vi "Продукты 2022.vi"() -> ()   [LabVIEW 2020]
uses:
  Control 2.ctl
panel:
  out "Array":T1[](array[typedef]) {"T" scale=-20.0..40.0; "Time Stamp" format="%<%2d/%2m/%4Y>T"}
  in  "Купить":bool
  in  "Покупаемый продукт":T1 {"T" scale=-20.0..40.0; "Time Stamp" format="%<%2d/%2m/%4Y>T"}
  in  "stop":bool
  out "String":string
  in  "Добавить":bool
  in  "Добавляемый продукт":T1 {"T" scale=-20.0..40.0; "Time Stamp" format="%<%2d/%2m/%4Y>T"}
  # "Прибыль магазина"
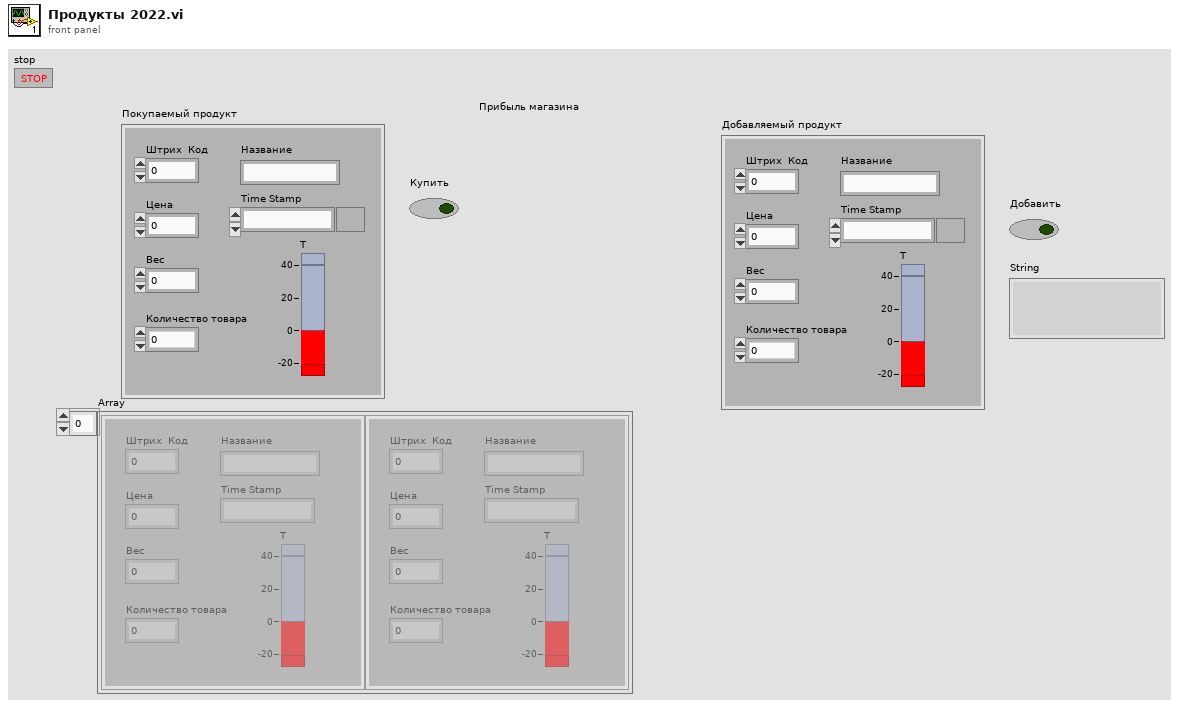
[diagram p1: front panel]
types:
  T1 = typedef "Control 2.ctl" = cluster{"Штрих  Код":dbl, "Цена":dbl, "Название":string, "Time Stamp":timestamp, "Вес":dbl, "T":dbl, "Количество товара":dbl}
  T2 = cluster{"Штрих  Код":dbl, "Цена":dbl, "Название":string, "Time Stamp":timestamp, "Вес":dbl, "T":dbl, "T 2":dbl}[]
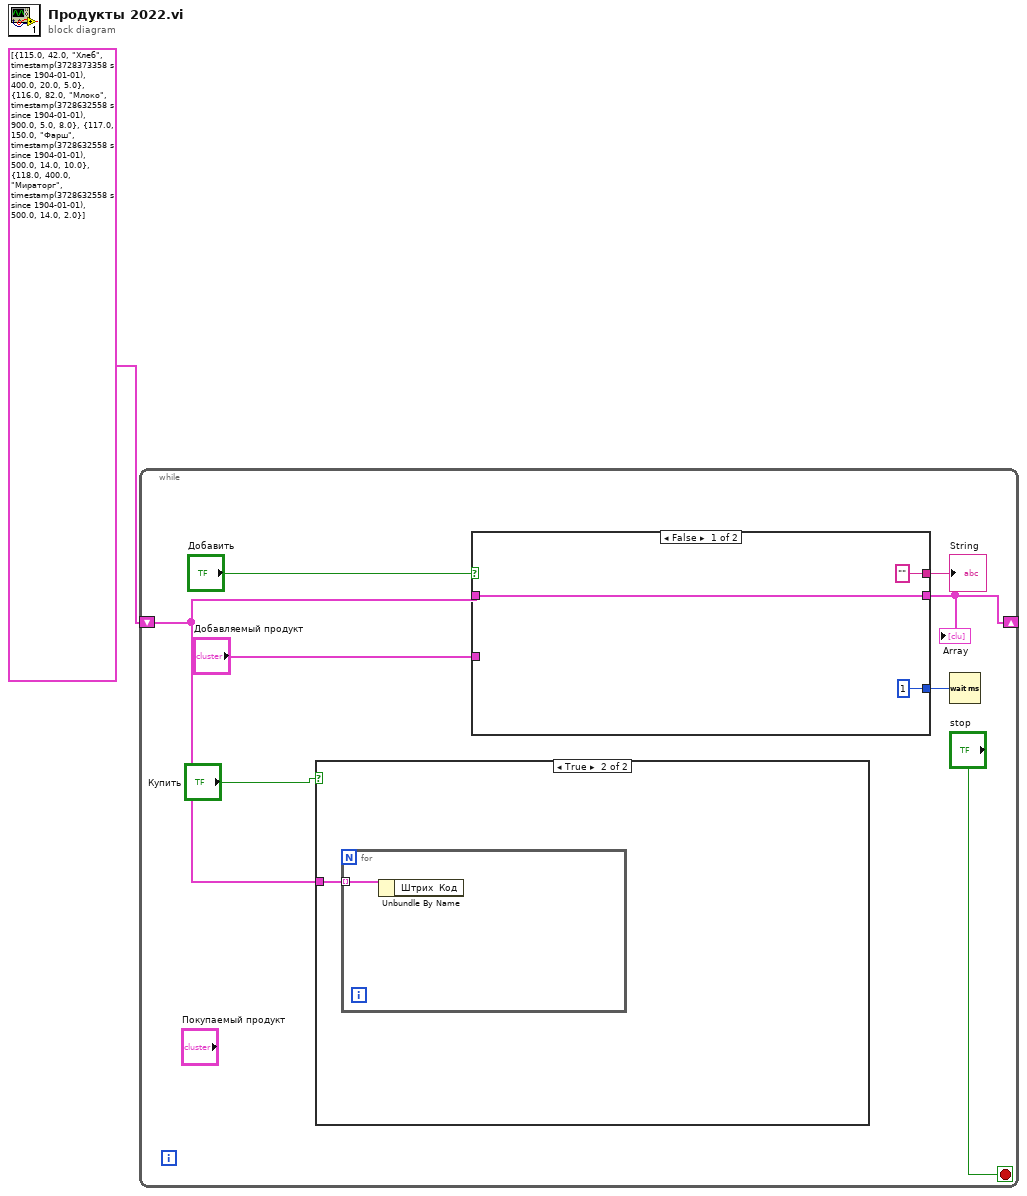
[diagram p0: block diagram]
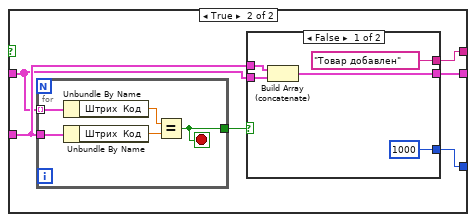
[diagram p3: hidden frame]
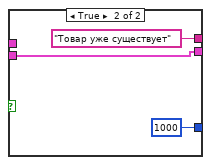
[diagram p4: hidden frame]
diagram:
  n1 = while {
    shift-right: [w2] -> _
    shift-left: T2 [{"Штрих  Код"=115.0, "Цена"=42.0, "Название"="Хлеб", "Time Stamp"=timestamp(3728373358.5762897 s since 1904-01-01), "Вес"=400.0, "T"=20.0, "T 2"=5.0}, {"Штрих  Код"=116.0, "Цена"=82.0, "Название"="Млоко", "Time Stamp"=timestamp(3728632558.5762897 s since 1904-01-01), "Вес"=900.0, "T"=5.0, "T 2"=8.0}, {"Штрих  Код"=117.0, "Цена"=150.0, "Название"="Фарш", "Time Stamp"=timestamp(3728632558.5762897 s since 1904-01-01), "Вес"=500.0, "T"=14.0, "T 2"=10.0}, {"Штрих  Код"=118.0, "Цена"=400.0, "Название"="Мираторг", "Time Stamp"=timestamp(3728632558.5762897 s since 1904-01-01), "Вес"=500.0, "T"=14.0, "T 2"=2.0}] -> [w3]
    stop <- "stop" stop-if-true
    n2 = case shown="True" "Купить" {
      tunnel: w3 -> [_ w10]
      frame False {
      }
      frame True {
        n3 = for {
          tunnel: w10 -> [w11] mode=indexing
          n4 = Unbundle By Name(w11) -> ()  [unwired: 1 out]
        }
      }
    }
    n5 = case shown="False" "Добавить" {
      tunnel: "Добавляемый продукт" -> [_ w16]
      tunnel: w3 -> [w12 w15]
      tunnel: [w12 w17] -> w2
      tunnel: ["" w19] -> w7
      tunnel: [u32 1 ("milliseconds to wait") w18] -> w6
      frame False {
      }
      frame True {
        n6 = for {
          tunnel: w16 -> [w33]
          tunnel: [w32] -> w20
          tunnel: w15 -> [w31] mode=indexing
          stop <- w32 stop-if-true
          n7 = Unbundle By Name(w31) -> ("Штрих  Код"=w30:dbl)
          n8 = Unbundle By Name(w33) -> ("Штрих  Код"=w29:dbl)
          n9 = Equal?(x=w30, y=w29) -> (x = y?=w32:bool)
        }
        n10 = case shown="False" w20 {
          tunnel: ["Товар добавлен" "Товар уже существует"] -> w19
          tunnel: [u32 1000 ("milliseconds to wait") u32 1000 ("milliseconds to wait")] -> w18
          tunnel: [w23 w26] -> w17
          tunnel: w16 -> [w22 _]
          tunnel: w15 -> [w21 w26]
          frame False {
            n11 = Build Array (concatenate)(w22, w21) -> (w23:T1[])
          }
          frame True {
          }
        }
      }
    }
    "String" <- w7
    "Array" <- w2
    n12 = Wait (ms)(milliseconds to wait=w6) -> ()  [unwired: 1 out]
  }
